vi "Get settings chain.vi"(8 "error in (no error)":errorcluster, 11 "TemplateBase in":refnum<class "Cobolt.lvclass">) -> (0 "error out":errorcluster, 1 "class name":string[](array[string]), 2 "settings":variant[](array[variant]), 3 "TemplateBase out":refnum<class "Cobolt.lvclass">)   [LabVIEW 2012, in "Cobolt.lvclass"]
doc: "Returns an array of variants containing the settings clusters of each class in the inheritance chain (lowest child class first), together with an array of all class names in the inheritance chain.\n\nFor classes without settings cluster, the settings chain contains empty variants."
uses:
  Cobolt.lvclass
  <vilib>/Distrio/Murmex/Murmex/Murmex.lvclass
  Cobolt.lvclass/Cobolt.ctl
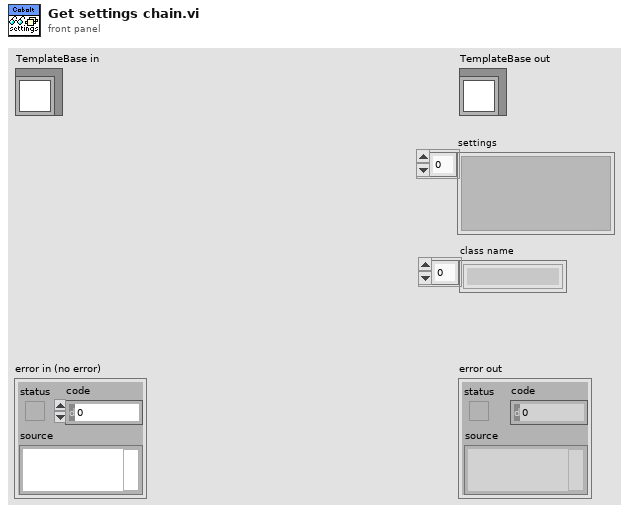
[diagram p1: front panel]
types:
  T1 = typedef "Cobolt.lvclass/settings_cluster.ctl" = cluster{"Power":dbl[unit], "Shutter":bool}
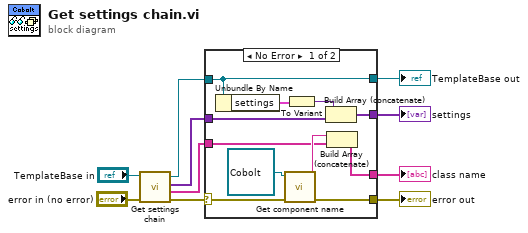
[diagram p0: block diagram]
diagram:
  n1 = call-parent "Get settings chain.vi"("error in (no error)"="error in (no error)", "MurmexBase in"="TemplateBase in") -> ("error out"=w8:errorcluster, "class name"=w1:string[], "settings"=w7:variant[], "MurmexBase out"=w6:refnum<class "Cobolt.lvclass">)  [unwired: 6 in]
  n2 = case shown="No Error" w8 {
    selector: w8 -> [w19 w25]
    tunnel: w1 -> [w18 w24]
    tunnel: w7 -> [w16 w23]
    tunnel: w6 -> [w14 w22]
    tunnel: [w14 w22] -> w5
    tunnel: [w13 w23] -> w4
    tunnel: [w12 w24] -> w3
    tunnel: [w11 w25] -> w2
    frame No Error {
      n3 = Unbundle By Name(w14) -> ("settings"=w20:T1)
      n4 = call <vilib>:"Get component name.vi"("error in (no error)"=w19, "Murmex in"=refnum<class "Cobolt.lvclass"> refnum ("Cobolt")) -> ("error out"=w11:errorcluster, "component name"=w21:string)  [unwired: 7 in, 1 out]
      n5 = To Variant(anything=w20) -> (Variant=w15:variant)
      n6 = Build Array (concatenate)(w15, w16) -> (w13:variant[])
      n7 = Build Array (concatenate)(w21, w18) -> (w12:string[])
    }
    frame Error {
    }
  }
  "error out" <- w2
  "TemplateBase out" <- w5
  "settings" <- w4
  "class name" <- w3
